vi "Get System Name.vi"(8 "error in (no error)":errorcluster, 11 "Trace Listener in":refnum<class "Trace Listener.lvclass">) -> (0 "error out":errorcluster, 2 "System Name":string, 3 "Trace Listener out":refnum<class "Trace Listener.lvclass">)   [LabVIEW 2014, in "Robot Actor Framework.lvlib" / "Trace.lvlib" / "Trace Listener.lvclass"]
uses:
  Trace Listener.lvclass
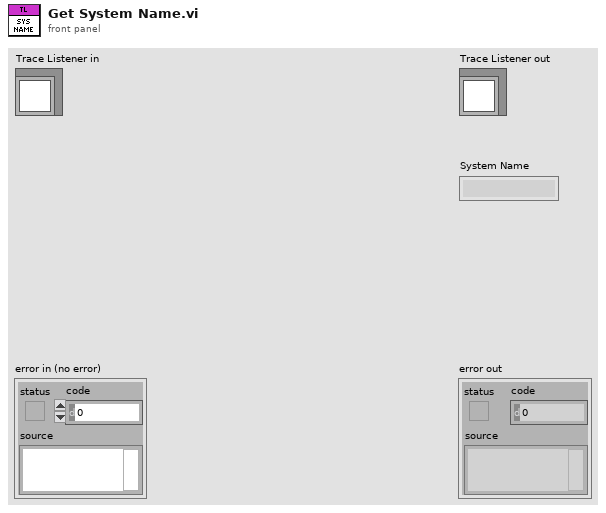
[diagram p1: front panel]
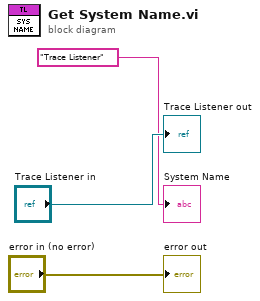
[diagram p0: block diagram]
diagram:
  "error out" <- "error in (no error)"
  "Trace Listener out" <- "Trace Listener in"
  "System Name" <- "Trace Listener"
